vi "Write StatusCode.vi"(8 "error in (no error)":errorcluster, 10 "StatusCode":u16, 11 "net-response in":refnum<class "net-response.lvclass">) -> (0 "error out":errorcluster, 3 "net-response out":refnum<class "net-response.lvclass">)   [LabVIEW 2020, in "net-response.lvclass"]
uses:
  net-response.lvclass
  net-response.lvclass/net-response.ctl
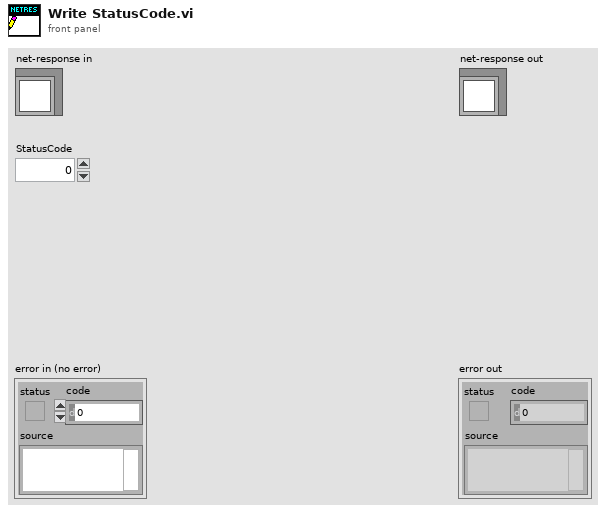
[diagram p1: front panel]
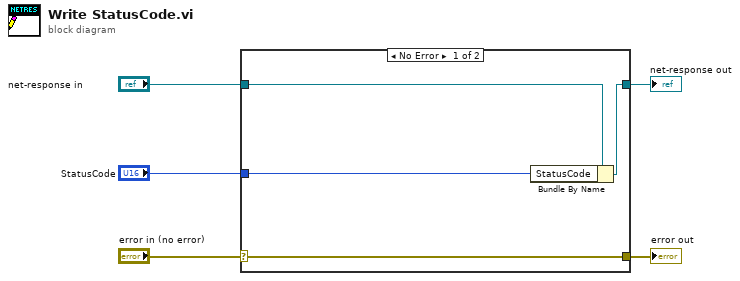
[diagram p0: block diagram]
diagram:
  n1 = case shown="No Error" "error in (no error)" {
    selector: "error in (no error)" -> [w9 w10]
    tunnel: [w9 w10] -> w4
    tunnel: [w7 w11] -> w2
    tunnel: "net-response in" -> [w8 w11]
    tunnel: "StatusCode" -> [w6 _]
    frame No Error {
      n2 = Bundle By Name(cluster=w8, "StatusCode"=w6) -> (w7:refnum<class "net-response.lvclass">)
    }
    frame Error {
    }
  }
  "error out" <- w4
  "net-response out" <- w2
